vi "Right Rocket Double Front Level 1 and 2.vi"(11 "Level 1? (F)":bool) -> ()   [LabVIEW 2018]
uses:
  Auton Kill Switch.vi
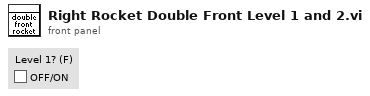
[diagram p1: front panel]
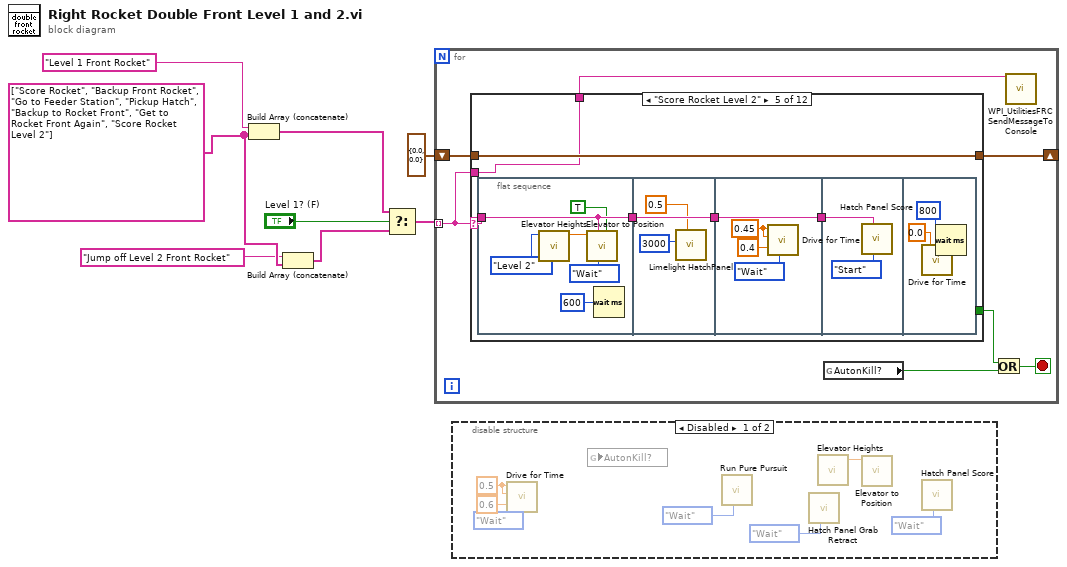
[diagram p0: block diagram]
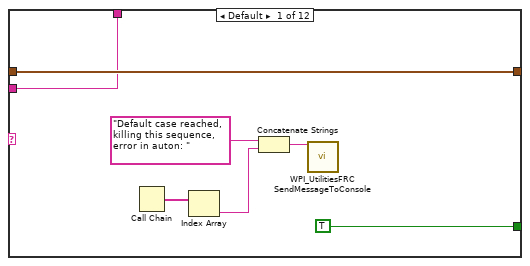
[diagram p3: hidden frame]
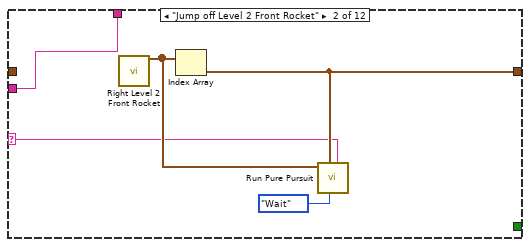
[diagram p4: hidden frame]
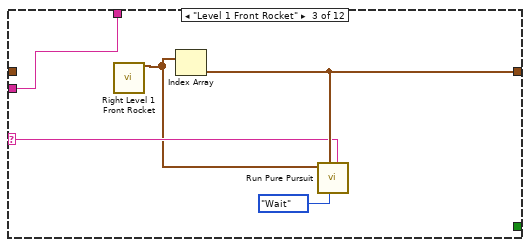
[diagram p5: hidden frame]
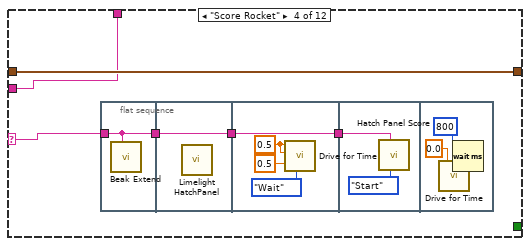
[diagram p6: hidden frame]
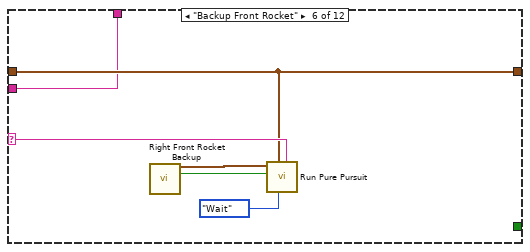
[diagram p7: hidden frame]
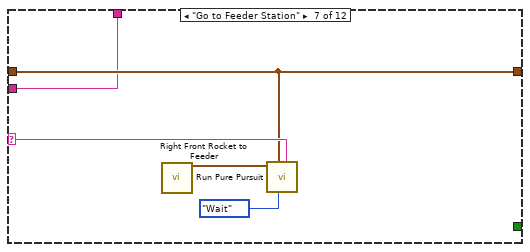
[diagram p8: hidden frame]
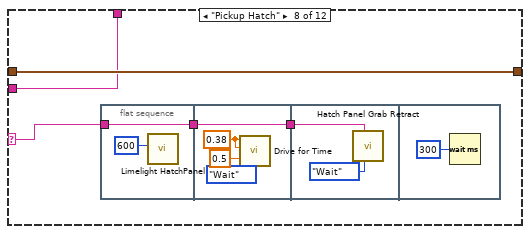
[diagram p9: hidden frame]
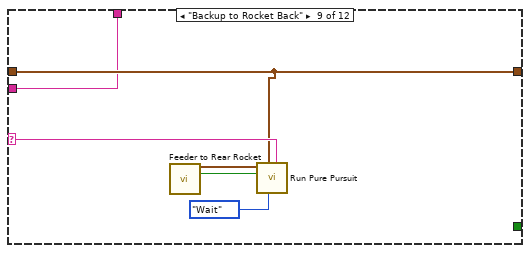
[diagram p10: hidden frame]
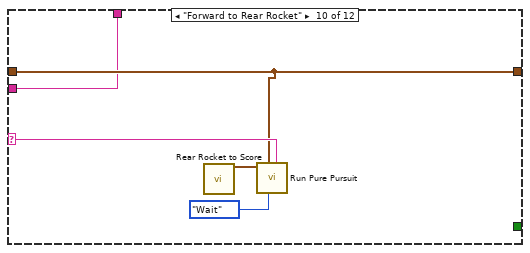
[diagram p11: hidden frame]
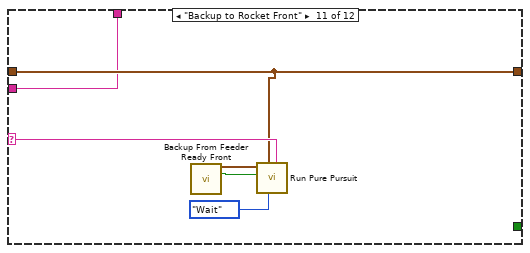
[diagram p12: hidden frame]
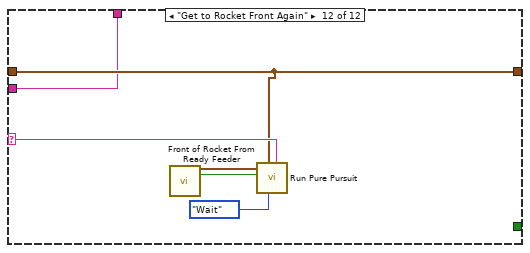
[diagram p13: hidden frame]
diagram:
  w6 = string[] ["Score Rocket", "Backup Front Rocket", "Go to Feeder Station", "Pickup Hatch", "Backup to Rocket Front", "Get to Rocket Front Again", "Score Rocket Level 2"]
  n1 = Build Array (concatenate)("Level 1 Front Rocket", w6) -> (w2:string[])
  n2 = Build Array (concatenate)("Jump off Level 2 Front Rocket", w6) -> (w3:string[])
  n3 = Select(t=w2, s="Level 1? (F)", f=w3) -> (s? t:f=w1:string[])
  n4 = for {
    tunnel: w1 -> [w9] mode=indexing
    shift-right: [w14] -> _
    shift-left: cluster{"X":dbl, "Y":dbl} {"X"=0.0, "Y"=0.0} -> [w13]
    stop <- w12 stop-if-true
    n5 = case shown="\"Score Rocket Level 2\"" w9 {
      selector: w9 -> [_ w24 w30 w34 w50 w74 w81 w86 w101 w106 w112 w118]
      tunnel: [w21 w25 w31 w38 w54 w73 w80 w87 w100 w105 w111 w117] -> w14
      tunnel: w13 -> [w21 _ _ w38 w54 w73 w80 w87 w100 w105 w111 w117]
      tunnel: [TRUE _ _ _ _ _ _ _ _ _ _ _] -> w11
      tunnel: [w16 w23 w29 w33 w49 w72 w78 w85 w97 w103 w110 w116] -> w10
      tunnel: w9 -> [w16 w23 w29 w33 w49 w72 w78 w85 w97 w103 w110 w116]
      frame Default {
        n6 = Call Chain() -> (call chain=w20:string[])
        n7 = Index Array(array=w20) -> (element=w18:string)  [unwired: 1 in]
        n8 = Concatenate Strings("Default case reached, killing this sequence, error in auton: " ("Message"), w18) -> (w17:string)
        n9 = call <vilib>:"WPI_UtilitiesFRC SendMessageToConsole.vi"("Message"=w17) -> ()  [unwired: 14 in, 1 out]
      }
      frame "Jump off Level 2 Front Rocket" {
        n10 = call "Right Level 2 Front Rocket.vi"() -> ("path"=w26:cluster{"X":dbl, "Y":dbl}[])  [unwired: 14 in, 1 out]
        n11 = Index Array(array=w26) -> (element=w25:cluster{"X":dbl, "Y":dbl})  [unwired: 1 in]
        n12 = call "Run Pure Pursuit.vi"("Description"=w24, "Synchronication"=enum16{"Start", "Wait"}."Wait", "Auton Start Point"=w25, "Path"=w26) -> ()  [unwired: 7 in, 1 out]
      }
      frame "Level 1 Front Rocket" {
        n13 = call "Right Level 1 Front Rocket.vi"() -> ("path"=w28:cluster{"X":dbl, "Y":dbl}[])  [unwired: 14 in, 1 out]
        n14 = Index Array(array=w28) -> (element=w31:cluster{"X":dbl, "Y":dbl})  [unwired: 1 in]
        n15 = call "Run Pure Pursuit.vi"("Description"=w30, "Synchronication"=enum16{"Start", "Wait"}."Wait", "Auton Start Point"=w31, "Path"=w28) -> ()  [unwired: 7 in, 1 out]
      }
      frame "Score Rocket" {
        n16 = flat-sequence {
          tunnel: w34 -> [w39]
          tunnel: [w39] -> w37
          tunnel: [w40] -> w36
          tunnel: w37 -> [w40]
          tunnel: w36 -> [w44]
          tunnel: [w44] -> w35
          tunnel: w35 -> [w45]
          frame #0 {
            n17 = call "Beak Extend.vi"("Description"=w39) -> ()  [unwired: 10 in, 1 out]
          }
          frame #1 {
            n18 = call "Limelight HatchPanel.vi"() -> ()  [unwired: 10 in, 2 out]
          }
          frame #2 {
            w43 = 0.5 ("Left Speed")
            n19 = call "Drive for Time.vi"("Synchronization"=enum16{"Start", "Wait"}."Wait", "Seconds"=0.5, "Right Speed"=w43, "Left Speed"=w43) -> ()  [unwired: 6 in, 2 out]
          }
          frame #3 {
            n20 = call "Hatch Panel Score.vi"("Synchronization"=enum16{"Start", "Wait"}."Start", "Description"=w45) -> ()  [unwired: 9 in, 1 out]
          }
          frame #4 {
            w47 = 0.0 ("Left Speed")
            n21 = call "Drive for Time.vi"("Seconds"=w47, "Right Speed"=w47, "Left Speed"=w47) -> ()  [unwired: 7 in, 2 out]
            n22 = Wait (ms)(milliseconds to wait=u32 800) -> ()  [unwired: 1 out]
          }
        }
      }
      frame "Score Rocket Level 2" {
        n23 = flat-sequence {
          tunnel: w50 -> [w58]
          tunnel: [w58] -> w53
          tunnel: [w63] -> w52
          tunnel: w53 -> [w63]
          tunnel: w52 -> [w67]
          tunnel: [w67] -> w51
          tunnel: w51 -> [w68]
          frame #0 {
            n24 = call "Elevator Heights.vi"("Level"=enum16{"Level 1", "Level 2", "Level 3"}."Level 2") -> ("Height"=w57:dbl)  [unwired: 8 in, 2 out]
            n25 = call "Elevator to Position.vi"("Extend at end of travel? (F)"=TRUE, "Synchronization"=enum16{"Start", "Wait"}."Wait", "Description"=w58, "Elevator Height"=w57) -> ()  [unwired: 7 in, 1 out]
            n26 = Wait (ms)(milliseconds to wait=u32 600) -> ()  [unwired: 1 out]
          }
          frame #1 {
            n27 = call "Limelight HatchPanel.vi"("Max Speed"=0.5, "Max Time ms (2000)"=u32 3000) -> ()  [unwired: 8 in, 2 out]
          }
          frame #2 {
            w66 = 0.45 ("Left Speed")
            n28 = call "Drive for Time.vi"("Synchronization"=enum16{"Start", "Wait"}."Wait", "Seconds"=0.4, "Right Speed"=w66, "Left Speed"=w66) -> ()  [unwired: 6 in, 2 out]
          }
          frame #3 {
            n29 = call "Hatch Panel Score.vi"("Synchronization"=enum16{"Start", "Wait"}."Start", "Description"=w68) -> ()  [unwired: 9 in, 1 out]
          }
          frame #4 {
            w70 = 0.0 ("Left Speed")
            n30 = call "Drive for Time.vi"("Seconds"=w70, "Right Speed"=w70, "Left Speed"=w70) -> ()  [unwired: 7 in, 2 out]
            n31 = Wait (ms)(milliseconds to wait=u32 800) -> ()  [unwired: 1 out]
          }
        }
      }
      frame "Backup Front Rocket" {
        n32 = call "Right Front Rocket Backup.vi"() -> ("path"=w76:cluster{"X":dbl, "Y":dbl}[], "Reverse Path?"=w75:bool)  [unwired: 14 in]
        n33 = call "Run Pure Pursuit.vi"("Description"=w74, "Synchronication"=enum16{"Start", "Wait"}."Wait", "Auton Start Point"=w73, "Reverse? (F)"=w75, "Path"=w76) -> ()  [unwired: 6 in, 1 out]
      }
      frame "Go to Feeder Station" {
        n34 = call "Right Front Rocket to Feeder.vi"() -> ("path"=w79:cluster{"X":dbl, "Y":dbl}[])  [unwired: 14 in, 1 out]
        n35 = call "Run Pure Pursuit.vi"("Description"=w81, "Synchronication"=enum16{"Start", "Wait"}."Wait", "Auton Start Point"=w80, "Path"=w79) -> ()  [unwired: 7 in, 1 out]
      }
      frame "Pickup Hatch" {
        n36 = flat-sequence {
          tunnel: w86 -> [w89]
          tunnel: [w89] -> w83
          tunnel: [w93] -> w84
          tunnel: w83 -> [w93]
          tunnel: w84 -> [w94]
          frame #0 {
            n37 = call "Limelight HatchPanel.vi"("Max Time ms (2000)"=u32 600) -> ()  [unwired: 9 in, 2 out]
          }
          frame #1 {
            w92 = 0.38 ("Left Speed")
            n38 = call "Drive for Time.vi"("Synchronization"=enum16{"Start", "Wait"}."Wait", "Seconds"=0.5, "Right Speed"=w92, "Left Speed"=w92) -> ()  [unwired: 6 in, 2 out]
          }
          frame #2 {
            n39 = call "Hatch Panel Grab Retract.vi"("Synchronization"=enum16{"Start", "Wait"}."Wait", "Description"=w94) -> ()  [unwired: 9 in, 1 out]
          }
          frame #3 {
            n40 = Wait (ms)(milliseconds to wait=u32 300) -> ()  [unwired: 1 out]
          }
        }
      }
      frame "Backup to Rocket Back" {
        n41 = call "Feeder to Rear Rocket.vi"() -> ("path"=w99:cluster{"X":dbl, "Y":dbl}[], "Reverse Path?"=w98:bool)  [unwired: 14 in]
        n42 = call "Run Pure Pursuit.vi"("Description"=w101, "Synchronication"=enum16{"Start", "Wait"}."Wait", "Auton Start Point"=w100, "Reverse? (F)"=w98, "Path"=w99) -> ()  [unwired: 6 in, 1 out]
      }
      frame "Forward to Rear Rocket" {
        n43 = call "Rear Rocket to Score.vi"() -> ("path"=w104:cluster{"X":dbl, "Y":dbl}[])  [unwired: 14 in, 1 out]
        n44 = call "Run Pure Pursuit.vi"("Description"=w106, "Synchronication"=enum16{"Start", "Wait"}."Wait", "Auton Start Point"=w105, "Path"=w104) -> ()  [unwired: 7 in, 1 out]
      }
      frame "Backup to Rocket Front" {
        n45 = call "Backup From Feeder Ready Front.vi"() -> ("path"=w109:cluster{"X":dbl, "Y":dbl}[], "Reverse Path?"=w108:bool)  [unwired: 14 in]
        n46 = call "Run Pure Pursuit.vi"("Description"=w112, "Synchronication"=enum16{"Start", "Wait"}."Wait", "Auton Start Point"=w111, "Reverse? (F)"=w108, "Path"=w109) -> ()  [unwired: 6 in, 1 out]
      }
      frame "Get to Rocket Front Again" {
        n47 = call "Front of Rocket From Ready Feeder.vi"() -> ("path"=w114:cluster{"X":dbl, "Y":dbl}[], "Reverse Path?"=w115:bool)  [unwired: 14 in]
        n48 = call "Run Pure Pursuit.vi"("Description"=w118, "Synchronication"=enum16{"Start", "Wait"}."Wait", "Auton Start Point"=w117, "Reverse? (F)"=w115, "Path"=w114) -> ()  [unwired: 6 in, 1 out]
      }
    }
    n49 = global read "Auton Kill Switch.vi" "AutonKill?"() -> (w15:bool)
    n50 = Or(x=w11, y=w15) -> (x .or. y?=w12:bool)
    n51 = call <vilib>:"WPI_UtilitiesFRC SendMessageToConsole.vi"("Message"=w10) -> ()  [unwired: 14 in, 1 out]
  }
  n52 = disable-structure shown="Disabled" {
    frame Disabled {
      w120 = 0.5 ("Left Speed")
      n53 = call "Drive for Time.vi"("Synchronization"=enum16{"Start", "Wait"}."Wait", "Seconds"=0.6, "Right Speed"=w120, "Left Speed"=w120) -> ()  [unwired: 6 in, 2 out]
      n54 = global read "Auton Kill Switch.vi" "AutonKill?"() -> ()  [unwired: 1 in]
      n55 = call "Run Pure Pursuit.vi"("Synchronication"=enum16{"Start", "Wait"}."Wait") -> ()  [unwired: 10 in, 1 out]
      n56 = call "Hatch Panel Grab Retract.vi"("Synchronization"=enum16{"Start", "Wait"}."Wait") -> ()  [unwired: 10 in, 1 out]
      n57 = call "Elevator Heights.vi"() -> ("Height"=w125:dbl)  [unwired: 9 in, 2 out]
      n58 = call "Elevator to Position.vi"("Elevator Height"=w125) -> ()  [unwired: 10 in, 1 out]
      n59 = call "Hatch Panel Score.vi"("Synchronization"=enum16{"Start", "Wait"}."Wait") -> ()  [unwired: 10 in, 1 out]
    }
    frame Enabled {
    }
  }
